vi "set_on_off.vi"(8 "error in (no error)":errorcluster, 10 "On (T)/OFF (F)":bool, 11 "VISA resource name":refnum<visa-resource-name>) -> (0 "error out":errorcluster, 2 "On (T)/OFF (F) setting":bool, 3 "VISA resource name out":refnum<visa-resource-name>)   [LabVIEW 2018]
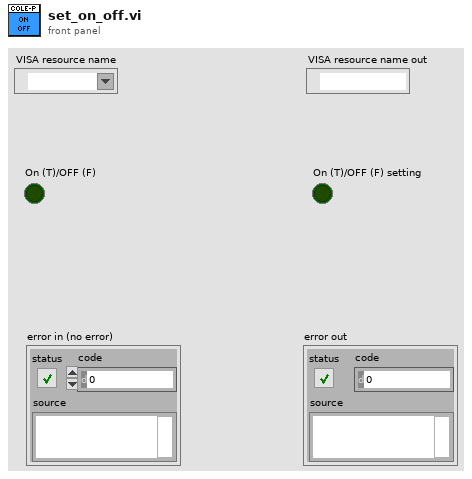
[diagram p1: front panel]
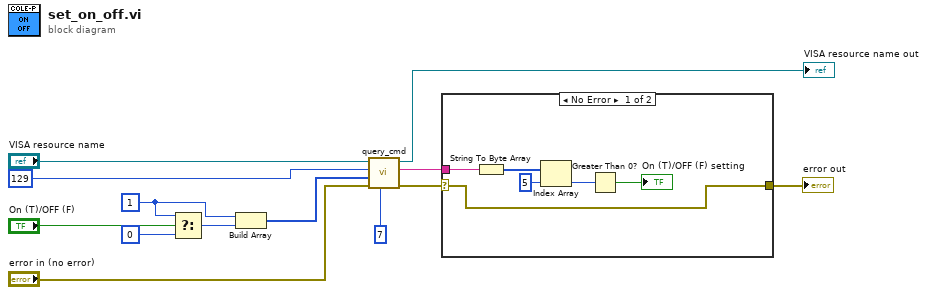
[diagram p0: block diagram]
diagram:
  w2 = u8 1
  n1 = Select(t=w2, s="On (T)/OFF (F)", f=u8 0) -> (s? t:f=w3:u8)
  n2 = Build Array(w2, w3) -> (w1:u8[])
  n3 = call "query_cmd.vi"("Number of bytes in response"=u32 7, "error in (no error)"="error in (no error)", "Data bytes"=w1, "Command byte"=u8 129, "VISA resource name"="VISA resource name") -> ("error out"=w7:errorcluster, "Response"=w8:string, "VISA resource name out"=→"VISA resource name out":refnum<visa-resource-name>)  [unwired: 4 in]
  n4 = case shown="No Error" w7 {
    selector: w7 -> [w19 w20]
    tunnel: w8 -> [w18 _]
    tunnel: [w19 w20] -> w6
    frame No Error {
      n5 = String To Byte Array(string=w18) -> (unsigned byte array=w17:u8[])
      n6 = Index Array(array=w17, index=5) -> (element=w15:u8)
      n7 = Greater Than 0?(x=w15) -> (x > 0?=→"On (T)/OFF (F) setting":bool)
    }
    frame Error {
    }
  }
  "error out" <- w6
